vi "Untethered Quadcopter.vi"() -> ()   [LabVIEW 2011]
uses:
  Controls/Motor dial ind.ctl
  <vilib>/addons/control/pid/pid.llb/PID Structure Conversion (DBL).vi
  <vilib>/addons/control/pid/pid.llb/PID (DBL).vi
  <vilib>/addons/control/pid/NI_PID_pid.lvlib
panel:
  in  "Framerate (FPS)":dbl=30.0 min=1.0 max=50.0 step=1.0 format="%#.6g"
  out "Position":cluster{"X":dbl, "Y":dbl, "Z":dbl}={"X"=0.0, "Y"=0.0, "Z"=-100.0}
  out "vy":picture
  in  "Turbulance":bool
  out "Angle (degrees)":dbl
  out "Angle":dbl(knob) scale=-30.0..30.0
  in  "Throttle":dbl(slide)=40.2 min=0.0 max=100.0 step=2.0 scale=0.0..100.0
  in  "PID gains":T1={"proportional gain (Kc)"=0.8, "Integral Gain"=25.0, "Derivative Gain"=0.004} {"Derivative Gain" format="%.3f"; "Integral Gain" format="%.3f"; "proportional gain (Kc)" format="%.3f"}
  in  "Control On/Off":bool=TRUE
  out "PID Out":dbl format="%0#4.1g"
  in  "Setpoint":dbl(knob) scale=-30.0..30.0
  out "Motor2":T2 scale=0.0..1000.0
  out "Motor4":T2 scale=0.0..1000.0
  in  "stop":bool
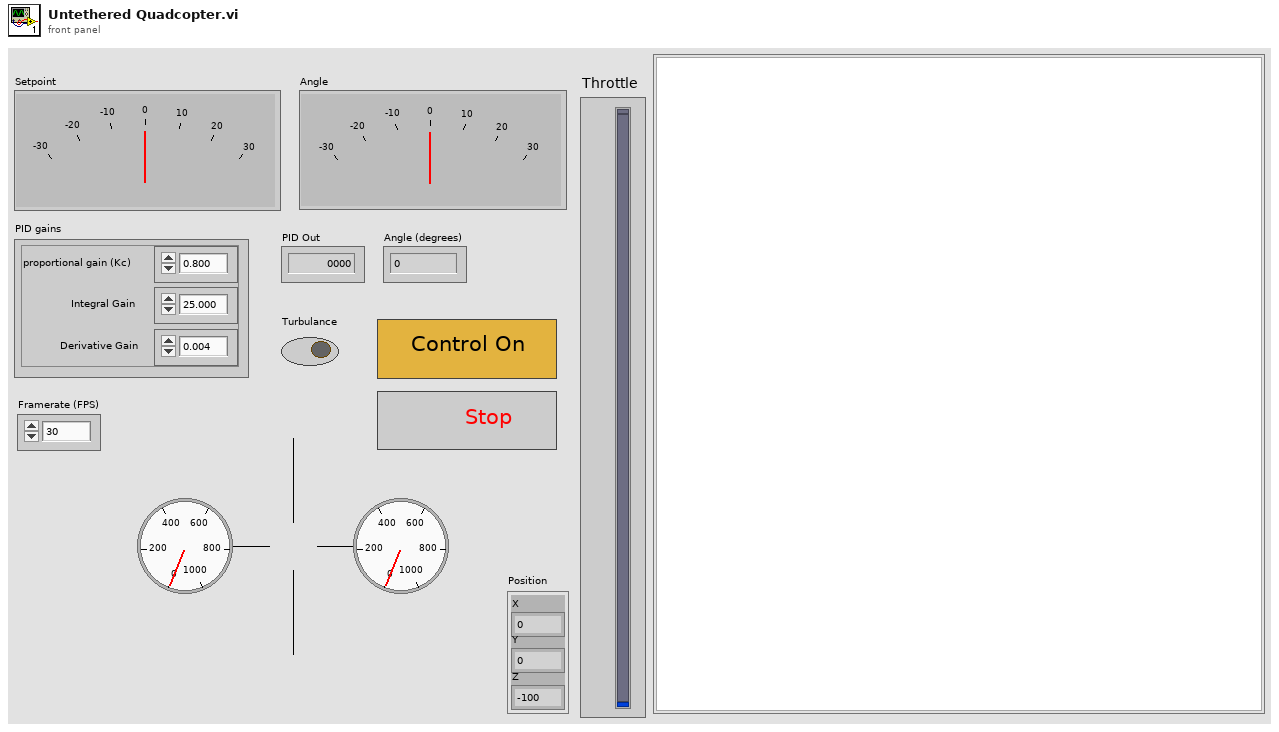
[diagram p1: front panel]
types:
  T1 = cluster{"proportional gain (Kc)":dbl, "Integral Gain":dbl, "Derivative Gain":dbl}
  T2 = typedef "Motor dial ind.ctl" = dbl
  T3 = cluster{"control":cluster{"rudder":i32, "aileron":i32}, "rotate":cluster{"pitch":dbl, "roll":dbl, "yaw":dbl}, "pos":cluster{"x":dbl, "y":dbl, "z":dbl}}
  T4 = enum16{"Academic (Standard)", "Parallel", "Series"}
  T5 = cluster{"proportional gain (Kc)":dbl, "integral time (Ti, min)":dbl, "derivative time (Td, min)":dbl}
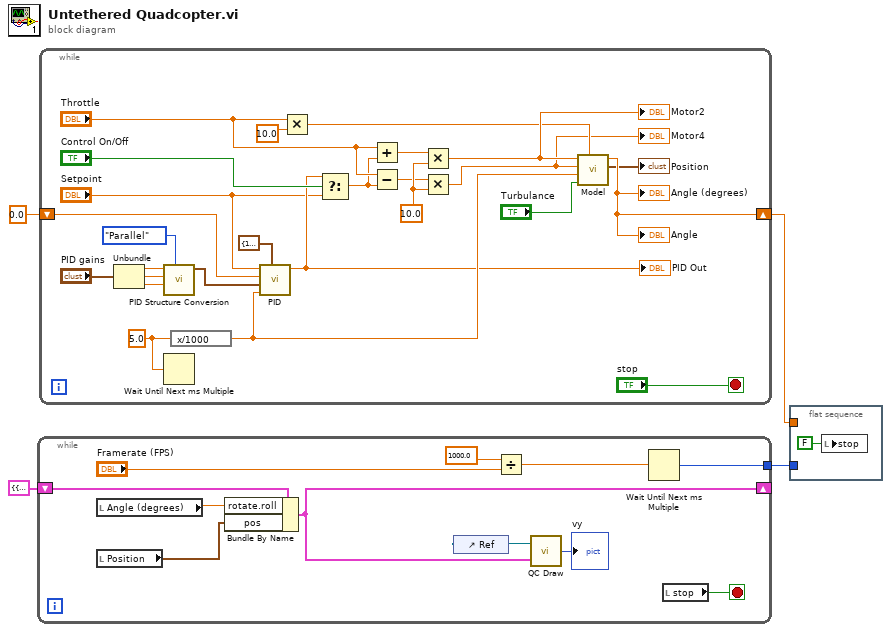
[diagram p0: block diagram]
diagram:
  n1 = while {
    tunnel: [w10] -> w2
    shift-right: [w9] -> _
    shift-left: T3 {"control"={"rudder"=0, "aileron"=0}, "rotate"={"pitch"=0.0, "roll"=0.0, "yaw"=0.0}, "pos"={"x"=0.0, "y"=0.0, "z"=1000.0}} ("steering") -> [w13]
    stop <- w11 stop-if-true
    n2 = local read "Angle (degrees)"() -> (w12:dbl)
    n3 = local read "Position"() -> (w8:cluster{"X":dbl, "Y":dbl, "Z":dbl})
    n4 = Bundle By Name(cluster=w13, "rotate.roll"=w12, "pos"=w8) -> (w9:T3)
    n5 = control-ref of="Ref"() -> (w15:refnum<vi>)
    n6 = Divide(x=1000.0, y="Framerate (FPS)") -> (x/y=w5:dbl)
    n7 = call "QC Draw.vi"("steering"=w9, "Picture Reference"=w15) -> ("picture out 2"=→"vy":picture)
    n8 = Wait Until Next ms Multiple(millisecond multiple=w5) -> (millisecond timer value=w10:u32)
    n9 = local read "stop"() -> (w11:bool)
  }
  n10 = while {
    shift-right: [w26] -> w1
    shift-left: 0.0 ("Angle (rads)") -> [w32]
    stop <- "stop" stop-if-true
    w34 = 5.0 ("dt (ms)")
    w40 = 10.0 ("y")
    n11 = Unbundle("PID gains") -> ("proportional gain (Kc)"=w38:dbl, "Integral Gain"=w37:dbl, "Derivative Gain"=w36:dbl)
    n12 = call-poly <vilib>:"PID Structure Conversion.vi"("PID structure"=T4."Parallel", "derivative"=w36, "integral"=w37, "proportional"=w38) -> ("PID gains"=w35:T5)  [unwired: 7 in]
    n13 = Wait Until Next ms Multiple(millisecond multiple=w34) -> ()  [unwired: 1 out]
    n14 = expression code="x/1000"(w34) -> (w31:dbl)
    n15 = call-poly <vilib>:"PID.vi"("output range"=cluster{"output high":dbl, "output low":dbl} {"output high"=100.0, "output low"=-100.0}, "dt (s)"=w31, "PID gains"=w35, "process variable"=w32, "setpoint"="Setpoint") -> ("output"=w18:dbl)  [unwired: 5 in, 1 out]
    "PID Out" <- w18
    n16 = Multiply(x="Throttle", y=10.0) -> (x*y=w23:dbl)
    n17 = Select(t=w18, s="Control On/Off", f="Setpoint") -> (s? t:f=w20:dbl)
    n18 = Add(x="Throttle", y=w20) -> (x+y=w30:dbl)
    n19 = Subtract(x="Throttle", y=w20) -> (x-y=w29:dbl)
    n20 = Multiply(x=w30, y=w40) -> (x*y=w28:dbl)
    "Motor2" <- w28
    n21 = Multiply(x=w29, y=w40) -> (x*y=w16:dbl)
    "Motor4" <- w16
    n22 = call "Model.vi"("Throttle"=w23, "Turbulance"="Turbulance", "dt (s)"=w31, "Motor 4"=w16, "Motor 2"=w28) -> ("Position"=→"Position":cluster{"X":dbl, "Y":dbl, "Z":dbl}, "Angle (degs)"=w26:dbl)  [unwired: 5 in]
    "Angle" <- w26
    "Angle (degrees)" <- w26
  }
  n23 = flat-sequence {
    tunnel: w2 -> [_]
    tunnel: w1 -> [_]
    frame #0 {
      n24 = local write "stop"(FALSE ("stop")) -> ()
    }
  }
